vi "main.vi"() -> ()   [LabVIEW 2020]
panel:
  out "x+y":dbl
  in  "y":dbl
  in  "x":dbl
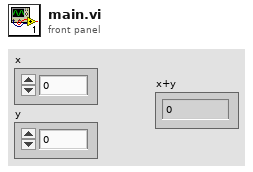
[diagram p1: front panel]
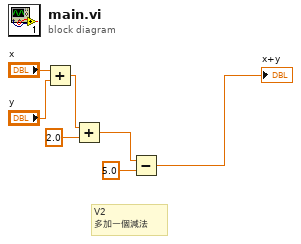
[diagram p0: block diagram]
diagram:
  # "V2\n多加一個減法"
  n1 = Add(x="x", y="y") -> (x+y=w5:dbl)
  n2 = Add(x=w5, y=2.0) -> (x+y=w2:dbl)
  n3 = Subtract(x=w2, y=5.0) -> (x-y=→"x+y":dbl)
